vi "Agilent 66XX Series Pause.vi"(0 "VISA resource name":refnum<visa-resource-name>, 7 "Pause(3000 ms)":u32=3000, 11 "error in (no error)":errorcluster) -> (15 "error out":errorcluster)   [LabVIEW 2012]
doc: "This VI illustrates how the instrument driver can be utilized to output saved parameters at a fixed time interval."
uses:
  <instrlib>/Agilent 66XX Series/Agilent 66XX Series.lvlib
panel:
  # "© 2005 National Instruments.  ALL RIGHTS RESERVED."
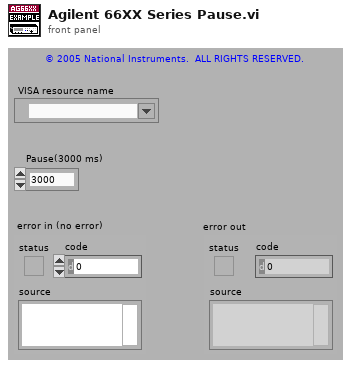
[diagram p1: front panel]
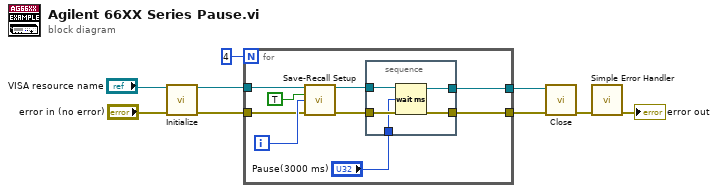
[diagram p0: block diagram]
diagram:
  n1 = call <instrlib>:"Initialize.vi"("VISA resource name"="VISA resource name", "error in (no error)"="error in (no error)") -> ("VISA resource name out"=w5:refnum<visa-resource-name>, "error out"=w6:errorcluster)  [unwired: 12 in]
  n2 = for {
    N: 4 -> [_]
    tunnel: w5 -> [w16]
    tunnel: w6 -> [w15]
    tunnel: [w11] -> w4
    tunnel: [w10] -> w3
    i -> [w18]
    n3 = call <instrlib>:"Save-Recall Setup.vi"("VISA resource name"=w16, "Mode(F:Save)"=TRUE, "Address (0)"=w18, "error in (no error)"=w15) -> ("VISA resource name out"=w13:refnum<visa-resource-name>, "error out"=w14:errorcluster)  [unwired: 10 in]
    n4 = stacked-sequence {
      tunnel: w14 -> [w21]
      tunnel: [w21] -> w10
      tunnel: w13 -> [w20]
      tunnel: [w20] -> w11
      tunnel: "Pause(3000 ms)" -> [w19]
      frame #0 {
        n5 = Wait (ms)(milliseconds to wait=w19) -> ()  [unwired: 1 out]
      }
    }
  }
  n6 = call <instrlib>:"Close.vi"("VISA resource name"=w4, "error in (no error)"=w3) -> ("error out"=w2:errorcluster)  [unwired: 13 in]
  n7 = call <vilib>:"Simple Error Handler.vi"("error in (no error)"=w2) -> ("error out"=→"error out":errorcluster)  [unwired: 4 in, 4 out]
